vi "Initialize.vi"(8 "error in (no error)":errorcluster, 10 "Path":path, 11 "ParseXML in":refnum<class "ParseSVG.lvclass">) -> (0 "error out":errorcluster, 3 "ParseXML out":refnum<class "ParseSVG.lvclass">)   [LabVIEW 2019, in "ParseSVG.lvclass"]
uses:
  ParseSVG.lvclass
  ParseSVG.lvclass/ParseSVG.ctl
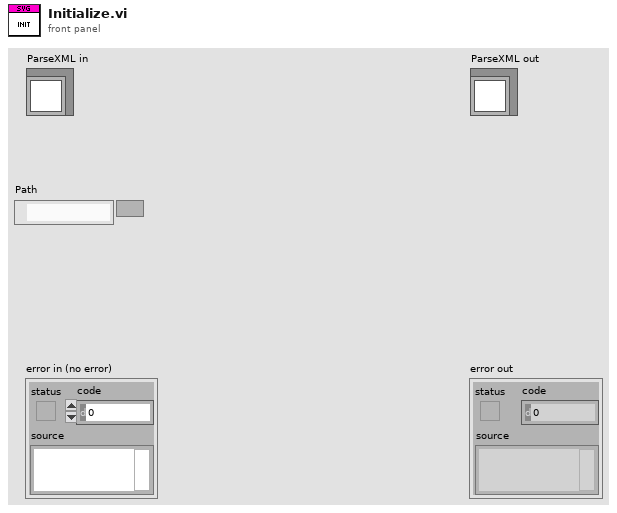
[diagram p1: front panel]
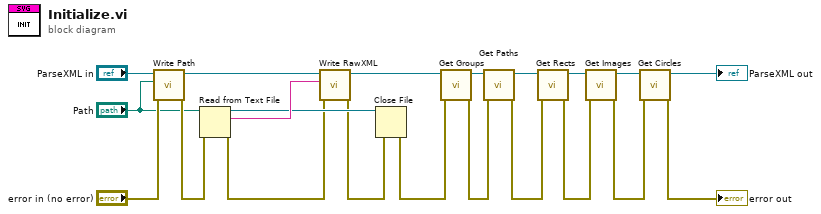
[diagram p0: block diagram]
diagram:
  n1 = call-dynamic "Write Path.vi"("error in (no error)"="error in (no error)", "Path"="Path", "ParseSVG in"="ParseXML in") -> ("error out"=w6:errorcluster, "ParseSVG out"=w8:refnum<class "ParseSVG.lvclass">)  [unwired: 7 in]
  n2 = Read from Text File(file (use dialog)="Path", error in=w6) -> (refnum out=w20:refnum<file>, text=w21:string, error out=w19:errorcluster)  [unwired: 2 in, 1 out]
  n3 = call "Write RawXML.vi"("error in (no error)"=w19, "RawXML"=w21, "ParseSVG.lvclass"=w8) -> ("error out"=w18:errorcluster, "ParseSVG.lvclass 2"=w4:refnum<class "ParseSVG.lvclass">)  [unwired: 7 in]
  n4 = Close File(refnum=w20, error in=w18) -> (error out=w2:errorcluster)  [unwired: 1 out]
  n5 = call "Get Groups.vi"("error in (no error)"=w2, "ParseSVG in"=w4) -> ("error out"=w1:errorcluster, "ParseSVG out"=w3:refnum<class "ParseSVG.lvclass">)  [unwired: 8 in]
  n6 = call "Get Paths.vi"("error in (no error)"=w1, "ParseXML in"=w3) -> ("error out"=w16:errorcluster, "ParseXML out"=w17:refnum<class "ParseSVG.lvclass">)  [unwired: 8 in]
  n7 = call "Get Rects.vi"("error in (no error)"=w16, "ParseSVG in"=w17) -> ("error out"=w14:errorcluster, "ParseSVG out"=w15:refnum<class "ParseSVG.lvclass">)  [unwired: 8 in]
  n8 = call "Get Images.vi"("error in (no error)"=w14, "ParseSVG in"=w15) -> ("error out"=w11:errorcluster, "ParseSVG out"=w13:refnum<class "ParseSVG.lvclass">)  [unwired: 8 in]
  n9 = call "Get Circles.vi"("error in (no error)"=w11, "ParseSVG in"=w13) -> ("error out"=→"error out":errorcluster, "ParseSVG out"=→"ParseXML out":refnum<class "ParseSVG.lvclass">)  [unwired: 8 in]
